vi "Untitled 3.vi"() -> ()   [LabVIEW 2015]
panel:
  out "done?":bool
  out "dummy var":dbl
  out "Elapsed Time (s)":dbl
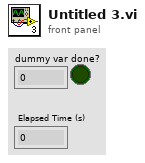
[diagram p1: front panel]
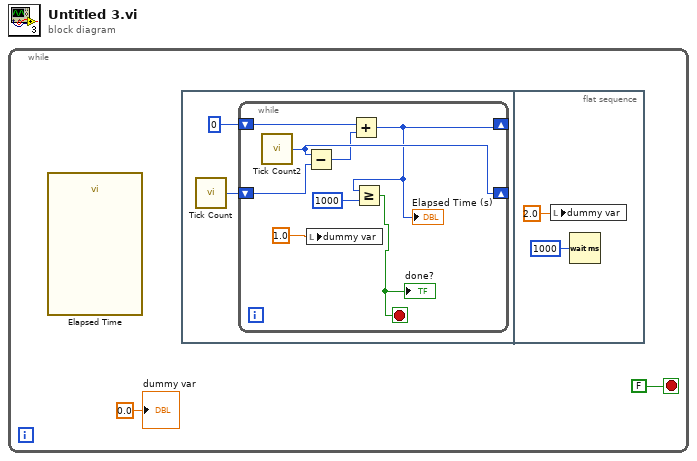
[diagram p0: block diagram]
diagram:
  n1 = while {
    stop <- FALSE stop-if-true
    n2 = call "Elapsed Time"() -> ()  [unwired: 12 in, 8 out]
    n3 = flat-sequence {
      frame #0 {
        n4 = call "Tick Count"() -> ("Tick Count(mSec)"=w4:u32)
        n5 = while {
          shift-right: [w9] -> _
          shift-left: w4 -> [w11]
          shift-right: [w5] -> _
          shift-left: 0 -> [w10]
          stop <- w6 stop-if-true
          n6 = call "Tick Count2"() -> ("Tick Count(mSec)"=w9:u32)
          n7 = Subtract(x=w9, y=w11) -> (x-y=w8:u32)
          n8 = local write "dummy var"(1.0) -> ()
          n9 = Add(x=w10, y=w8) -> (x+y=w5:u32)
          "Elapsed Time (s)" <- w5
          n10 = Greater Or Equal?(x=w5, y=u32 1000) -> (x >= y?=w6:bool)
          "done?" <- w6
        }
      }
      frame #1 {
        n11 = local write "dummy var"(2.0) -> ()
        n12 = Wait (ms)(milliseconds to wait=u32 1000) -> ()  [unwired: 1 out]
      }
    }
    "dummy var" <- 0.0
  }
